vi "Miernik.vi"() -> ()   [LabVIEW 2017]
uses:
  <vilib>/Instr/_visa.llb/VISA Configure Serial Port (Instr).vi
panel:
  out "bieżąca średnia PM 10":dbl
  in  "Plik do zapisu danych":path
  out "PM 10":string
  in  "stop":bool
  out "Natezenie":dbl(graph)
  out "Temperatura":dbl(graph)
  out "Wilgotnosc":dbl(graph)
  out "Wilgotność, temperatura i natężenie światła":string
  out "read buffer":string
  in  "Port szeregowy":refnum<visa-resource-name>="ASRL2::INSTR"
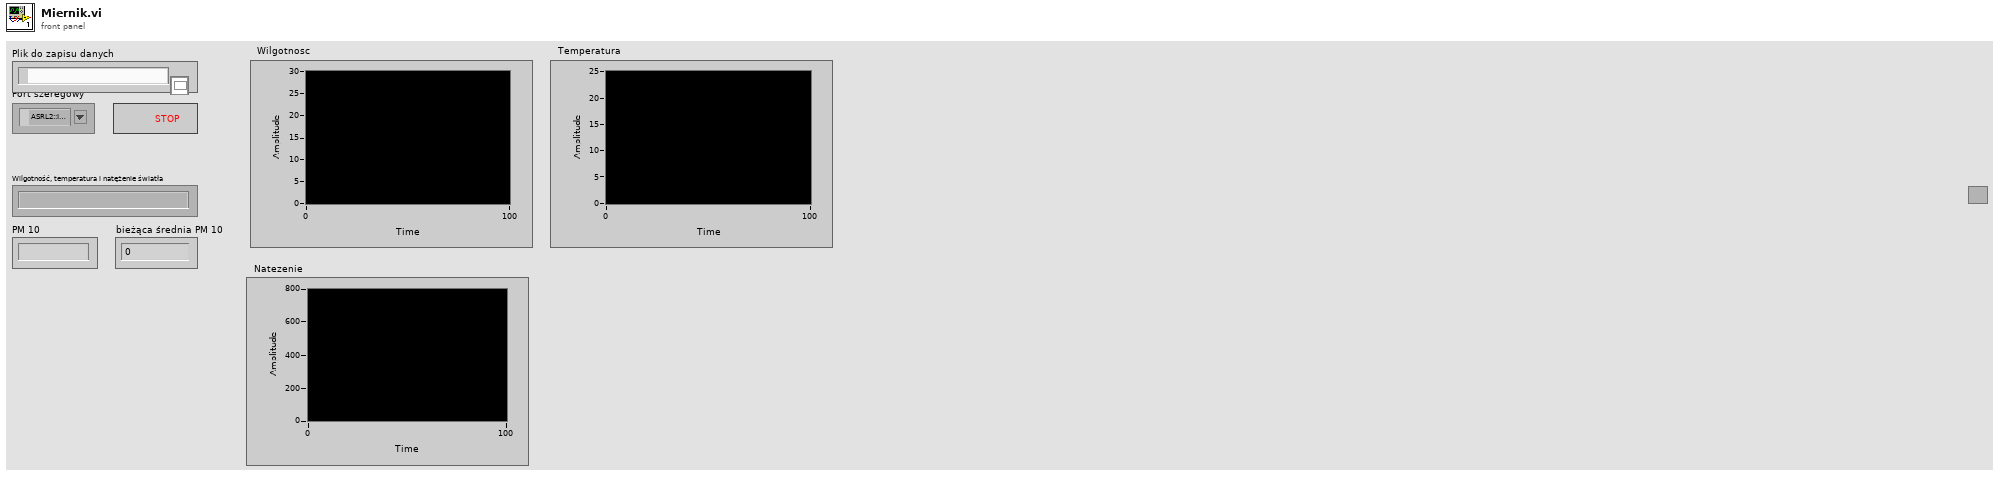
[diagram p1: front panel]
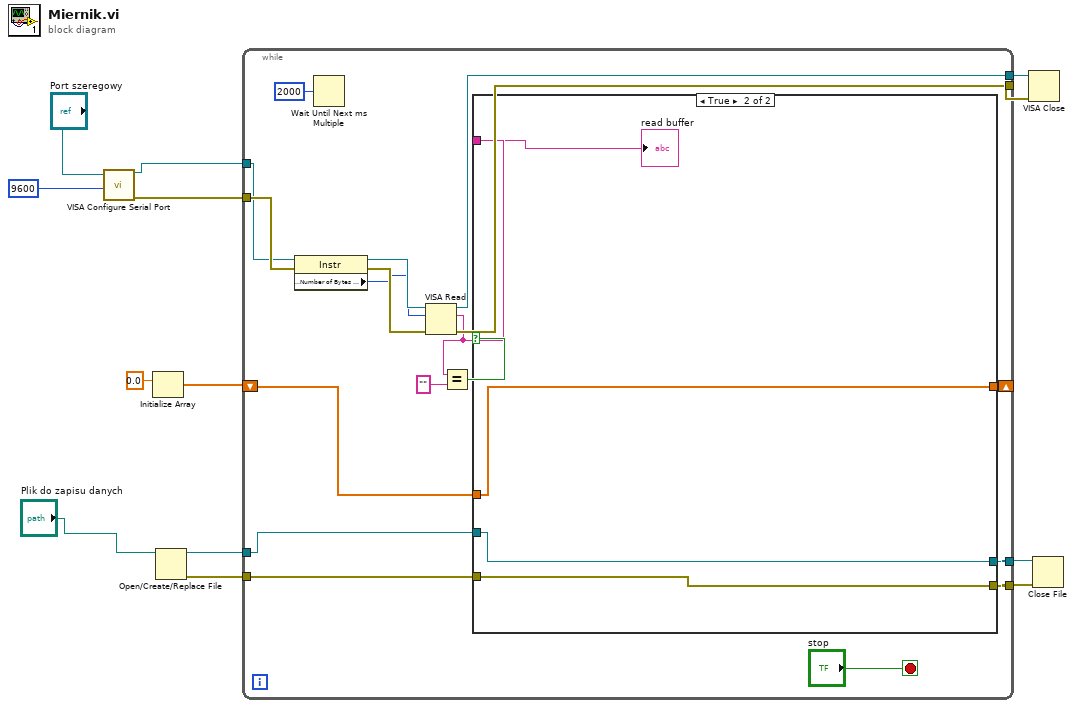
[diagram p0: block diagram]
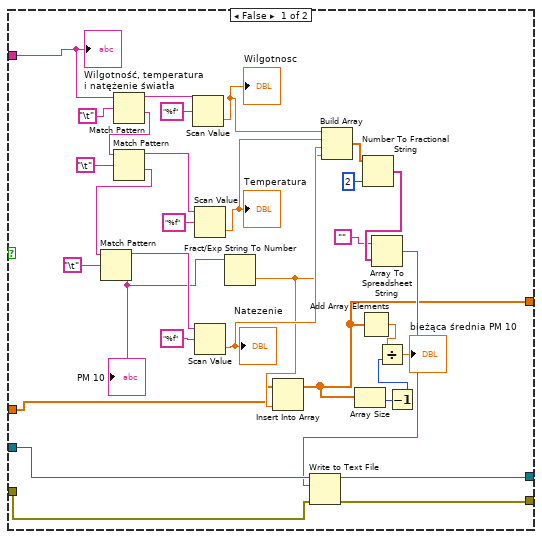
[diagram p2: hidden frame]
diagram:
  n1 = call-poly "VISA Configure Serial Port"("VISA resource name"="Port szeregowy", "baud rate (9600)"=u32 9600) -> ("VISA resource name out"=w11:refnum<visa-resource-name>, "error out"=w10:errorcluster)  [unwired: 12 in]
  n2 = Initialize Array(0.0 ("element")) -> (w2:dbl[])  [unwired: 1 in]
  n3 = Open/Create/Replace File(file path (use dialog)="Plik do zapisu danych") -> (refnum out=w7:refnum<file>, error out=w6:errorcluster)  [unwired: 5 in, 1 out]
  n4 = while {
    tunnel: w11 -> [w27]
    tunnel: w10 -> [w28]
    tunnel: [w23] -> w9
    tunnel: [w22] -> w8
    tunnel: w7 -> [w19]
    tunnel: w6 -> [w18]
    tunnel: [w17] -> w5
    tunnel: [w16] -> w4
    shift-right: [w14] -> _
    shift-left: w2 -> [w15]
    stop <- "stop" stop-if-true
    n5 = property class="Instr"(reference=w27, error in=w28) -> (reference out=w31:refnum<visa-resource-name>, error out=w30:errorcluster, "Serial Settings:Number of Bytes at Serial Port"=w29:u32)
    n6 = Wait Until Next ms Multiple(millisecond multiple=u32 2000) -> ()  [unwired: 1 out]
    n7 = VISA Read(VISA resource name=w31, byte count=w29, error in (no error)=w30) -> (VISA resource name out=w23:refnum<visa-resource-name>, read buffer=w21:string, error out=w22:errorcluster)  [unwired: 1 out]
    n8 = Equal?(x=w21, y="") -> (x = y?=w24:bool)
    n9 = case shown="True" w24 {
      tunnel: w21 -> [w58 w67]
      tunnel: w19 -> [w45 w66]
      tunnel: w18 -> [w48 w65]
      tunnel: [w47 w66] -> w17
      tunnel: [w46 w65] -> w16
      tunnel: w15 -> [w36 w64]
      tunnel: [w35 w64] -> w14
      frame False {
        n10 = Match Pattern(string=w58, regular expression="\t") -> (before substring=w62:string, after substring=w60:string)  [unwired: 1 in, 2 out]
        n11 = Match Pattern(string=w60, regular expression="\t") -> (before substring=w44:string, after substring=w42:string)  [unwired: 1 in, 2 out]
        n12 = Match Pattern(string=w42, regular expression="\t") -> (before substring=w41:string, after substring=w40:string)  [unwired: 1 in, 2 out]
        "PM 10" <- w40
        n13 = Scan Value(string=w62, format string="%f") -> (value=w55:dbl)  [unwired: 1 in, 1 out]
        "Wilgotnosc" <- w55
        n14 = Scan Value(string=w44, format string="%f") -> (value=w54:dbl)  [unwired: 1 in, 1 out]
        "Temperatura" <- w54
        n15 = Scan Value(string=w41, format string="%f") -> (value=w53:dbl)  [unwired: 1 in, 1 out]
        "Natezenie" <- w53
        n16 = Fract/Exp String To Number(string=w40) -> (number=w37:dbl)  [unwired: 3 in, 1 out]
        n17 = Insert Into Array(array=w36, new element=w37) -> (w35:dbl[])  [unwired: 1 in]
        n18 = Build Array(w55, w54, w53, w37) -> (w52:dbl[])
        n19 = Array Size(array=w35) -> (size(s)=w33:i32)
        n20 = Add Array Elements(numeric array=w35) -> (sum=w38:dbl)
        n21 = Number To Fractional String(number=w52, precision (6)=i16 2) -> (F-format string=w50:string[])  [unwired: 2 in]
        n22 = Array To Spreadsheet String(array=w50, 3:"") -> (spreadsheet string=w39:string)  [unwired: 1 in]
        n23 = Write to Text File(file (use dialog)=w45, text=w39, error in=w48) -> (refnum out=w47:refnum<file>, error out=w46:errorcluster)  [unwired: 1 in, 1 out]
        n24 = Decrement(x=w33) -> (x-1=w32:i32)
        n25 = Divide(x=w38, y=w32) -> (x/y=→"bieżąca średnia PM 10":dbl)
        "Wilgotność, temperatura i natężenie światła" <- w58
      }
      frame True {
        "read buffer" <- w67
      }
    }
  }
  n26 = VISA Close(VISA resource name=w9, error in (no error)=w8) -> ()  [unwired: 1 out]
  n27 = Close File(refnum=w5, error in=w4) -> ()  [unwired: 2 out]
